vi "read_init.vi"(8 "error in (no error)":errorcluster, 11 "MDS in":refnum<class "MDS.lvclass">) -> (0 "error out":errorcluster, 2 "init":dbl[](array[numeric]), 3 "MDS out":refnum<class "MDS.lvclass">)   [LabVIEW 2020, in "MDS.lvclass"]
uses:
  MDS.lvclass
  MDS.lvclass/MDS.ctl
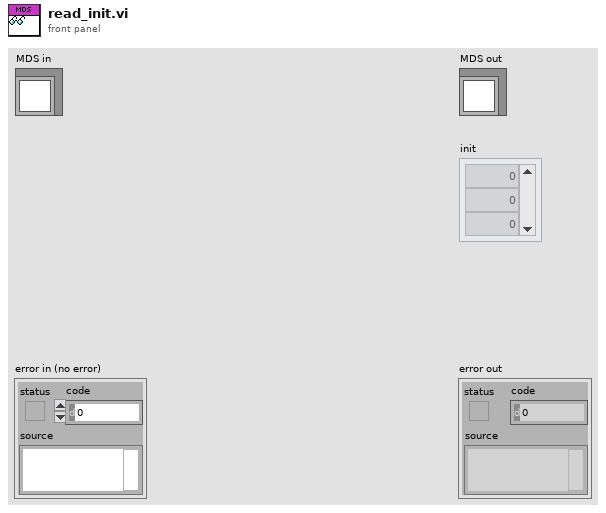
[diagram p1: front panel]
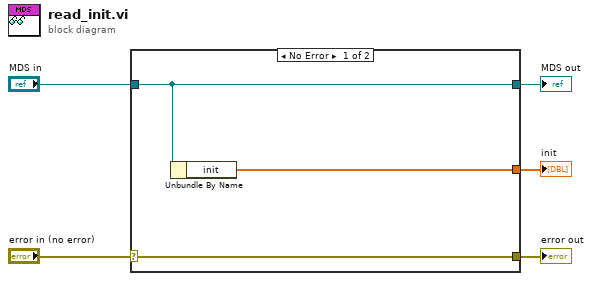
[diagram p0: block diagram]
diagram:
  n1 = case shown="No Error" "error in (no error)" {
    selector: "error in (no error)" -> [w8 w9]
    tunnel: [w8 w9] -> w4
    tunnel: [w7 w10] -> w2
    tunnel: "MDS in" -> [w7 w10]
    tunnel: [w6 _] -> w1
    frame No Error {
      n2 = Unbundle By Name(w7) -> ("init"=w6:dbl[])
    }
    frame Error {
    }
  }
  "error out" <- w4
  "MDS out" <- w2
  "init" <- w1
